vi "Untitled 2.vi"() -> ()   [LabVIEW 2015]
doc: "Krzysztof Cichy 16.10.2018"
panel:
  out "Warning":bool
  out "Warning Text":string
  in  "Min Temperature":dbl
  in  "Max Temperature":dbl
  in  "Current Temperature":dbl
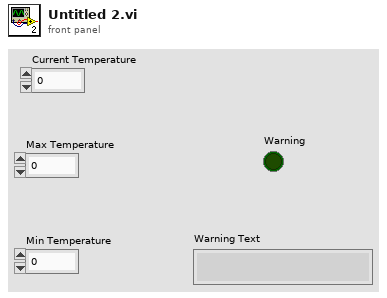
[diagram p1: front panel]
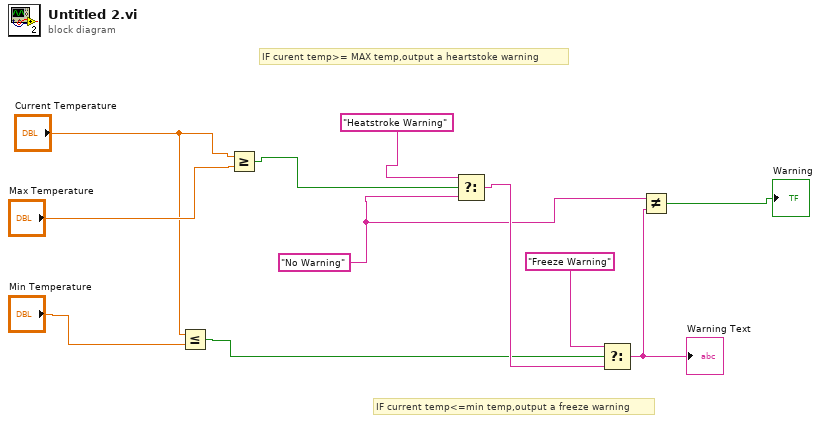
[diagram p0: block diagram]
diagram:
  w3 = "No Warning"
  # "IF current temp<=min temp,output a freeze warning"
  # "IF curent temp>= MAX temp,output a heartstoke warning"
  n1 = Less Or Equal?(x="Current Temperature", y="Min Temperature") -> (x <= y?=w4:bool)
  n2 = Greater Or Equal?(x="Current Temperature", y="Max Temperature") -> (x >= y?=w7:bool)
  n3 = Select(t="Heatstroke Warning", s=w7, f=w3) -> (s? t:f=w5:string)
  n4 = Select(t="Freeze Warning", s=w4, f=w5) -> (s? t:f=w1:string)
  "Warning Text" <- w1
  n5 = Not Equal?(x=w3, y=w1) -> (x != y?=→"Warning":bool)
